vi "Board Setup.vi"() -> (2 "Square[][]":refnum<class "Square.lvclass">[][](array[class]))   [LabVIEW 2015, in "SB SubVIs.lvlib"]
uses:
  SB SubVIs.lvlib
  Square/Square.lvclass
  Type Defs/Square Cluster.ctl
  Globals (private).vi
  Globals.vi
  Type Defs/SB Type Defs.lvlib
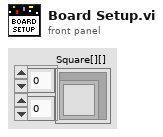
[diagram p1: front panel]
types:
  T1 = typedef "SB Type Defs.lvlib/Square Cluster.ctl" = cluster{"Attacked":bool, "Team":i32, "Next Turn":i32}
  T2 = cluster{"Color":u32, "Index":i32, "Status":string, "Stats":string}[]
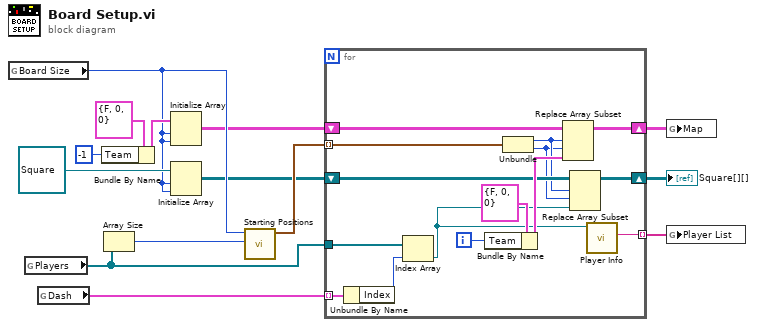
[diagram p0: block diagram]
diagram:
  n1 = global read "Globals (private).vi" "Board Size"() -> (w9:i32)
  n2 = global read "Globals (private).vi" "Players"() -> (w5:refnum<class "Square.lvclass">[])
  n3 = global read "Globals (private).vi" "Dash"() -> (w3:T2)
  n4 = Bundle By Name(cluster=T1 {"Attacked"=FALSE, "Team"=0, "Next Turn"=0} ("Cluster"), "Team"=-1) -> (w13:T1)
  n5 = Array Size(array=w5) -> (size(s)=w10:i32)
  n6 = Initialize Array(w13, w9, w9) -> (w8:T1[][])
  n7 = Initialize Array(refnum<class "Square.lvclass"> refnum ("element"), w9, w9) -> (w6:refnum<class "Square.lvclass">[][])
  n8 = call "Starting Positions.vi"("Player Count"=w10, "Size"=w9) -> ("Positions[]"=w7:cluster{i32, i32}[])  [unwired: 9 in]
  n9 = for {
    tunnel: w7 -> [w27] mode=indexing
    tunnel: w3 -> [w22] mode=indexing
    shift-right: [w28] -> w4
    shift-left: w8 -> [w29]
    tunnel: w5 -> [w24]
    tunnel: [w20] -> w2 mode=indexing
    shift-right: [w16] -> w1
    shift-left: w6 -> [w19]
    i -> [w21]
    n10 = Unbundle By Name(w22) -> ("Index"=w23:i32)
    n11 = Index Array(array=w24, index=w23) -> (element=w18:refnum<class "Square.lvclass">)
    n12 = Bundle By Name(cluster=T1 {"Attacked"=FALSE, "Team"=0, "Next Turn"=0} ("Cluster"), "Team"=w21) -> (w25:T1)
    n13 = Unbundle(w27) -> (w17:i32, w15:i32)
    n14 = Replace Array Subset(array=w29, new element=w25, index (row)=w17, index (col)=w15) -> (w28:T1[][])
    n15 = Replace Array Subset(array=w19, new element=w18, index (row)=w17, index (col)=w15) -> (w16:refnum<class "Square.lvclass">[][])
    n16 = call-dynamic "Player Info.vi"("Square in"=w18) -> ("Name"=w20:string)  [unwired: 7 in, 3 out]
  }
  "Square[][]" <- w1
  n17 = global write "Globals.vi" "Map"(w4) -> ()
  n18 = global write "Globals (private).vi" "Player List"(w2) -> ()
